vi "symmetry_transform_check_ROI.vi"(4 "error in (no error)":errorcluster, 5 "minimum size":i32, 6 "Optional Rectangle":i32[](array[numeric]), 7 "Image Src":T1) -> (0 "error out":errorcluster, 2 "ROI Out (x,y,w,h)":i32[](array[numeric]), 3 "Image Src Dup":T1)   [LabVIEW 2010]
uses:
  <vilib>/vision/Image Controls.llb/IMAQ Image.ctl
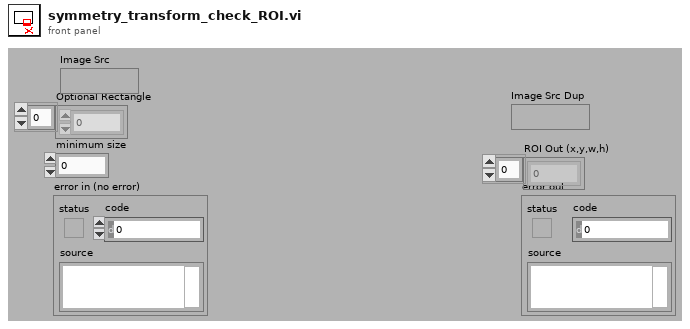
[diagram p1: front panel]
types:
  T1 = typedef "IMAQ Image.ctl" = refnum<image>
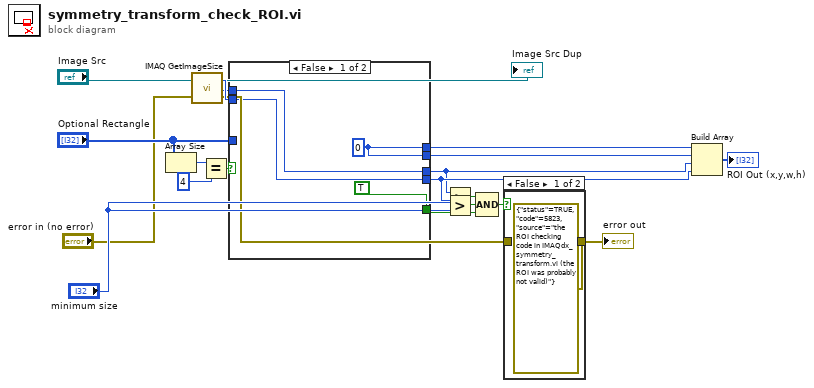
[diagram p0: block diagram]
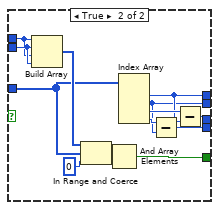
[diagram p3: hidden frame]
diagram:
  n1 = Array Size(array="Optional Rectangle") -> (size(s)=w10:i32)
  n2 = call "IMAQ GetImageSize"("Image"="Image Src", "error in (no error)"="error in (no error)") -> ("Y Resolution"=w15:i32, "X Resolution"=w14:i32, "error out"=w1:errorcluster)  [unwired: 2 out]
  n3 = Equal?(x=w10, y=4) -> (x = y?=w12:bool)
  n4 = case shown="False" w12 {
    tunnel: "Optional Rectangle" -> [_ w25]
    tunnel: w14 -> [w23 w36]
    tunnel: w15 -> [w22 w37]
    tunnel: [w24 w32] -> w7
    tunnel: [w24 w30] -> w6
    tunnel: [w23 w29] -> w4
    tunnel: [w22 w28] -> w5
    tunnel: [TRUE w26] -> w18
    frame False {
      w24 = 0 ("Y Resolution")
    }
    frame True {
      n5 = Build Array(w36, w37, w36, w37) -> (w35:i32[])
      n6 = In Range and Coerce(upper limit=w35, x=w25, lower limit=0 ("LineWidth(Pixels)")) -> (In Range?=w27:bool[])  [unwired: 1 out]
      n7 = And Array Elements(Boolean array=w27) -> (logical AND=w26:bool)
      n8 = Index Array(array=w25) -> (element #1=w32:i32, element #2=w30:i32, element #3=w33:i32, element #4=w31:i32)  [unwired: 4 in]
      n9 = Subtract(x=w31, y=w30) -> (x-y=w28:i32)
      n10 = Subtract(x=w33, y=w32) -> (x-y=w29:i32)
    }
  }
  n11 = Greater?(x=w4, y="minimum size") -> (0:w16:bool)
  n12 = Greater?(x=w5, y="minimum size") -> (0:w17:bool)
  n13 = Compound Arithmetic op=AND(w16, w17, w18) -> (w20:bool)
  n14 = case shown="False" w20 {
    tunnel: w1 -> [_ w39]
    tunnel: [errorcluster {"status"=TRUE, "code"=5823, "source"="the ROI checking code in IMAQdx_symmetry_transform.vi (the ROI was probably not valid)"} ("error in (no error)") w39] -> w19
    frame False {
    }
    frame True {
    }
  }
  "error out" <- w19
  n15 = Build Array(w7, w6, w4, w5) -> (→"ROI Out (x,y,w,h)":i32[])
  "Image Src Dup" <- "Image Src"
